vi "clear_buffers.vi"(8 "error in (no error)":errorcluster, 11 "DAQ_DL091205Readers in":refnum<class "DAQ_DL091205Readers.lvclass">) -> (0 "error out":errorcluster, 3 "DAQ_DL091205Readers out":refnum<class "DAQ_DL091205Readers.lvclass">)   [LabVIEW 2010, in "DAQ_DL091205Readers.lvclass"]
uses:
  DAQ_DL091205Readers.lvclass
  DAQ_DL090211Scaffold/DAQ_DL090211Scaffold/DAQ_DL090211Scaffold.lvclass
  DAQ_DL091205Readers.lvclass/DAQ_DL091205Readers.ctl
  SignalReader/GenericSignalReader/GenericSignalReader/GenericSignalReader.lvclass
  common/classes/ErrorController/ErrorController/class_data.vi
  common/classes/ErrorController/ErrorController/ErrorController.lvclass
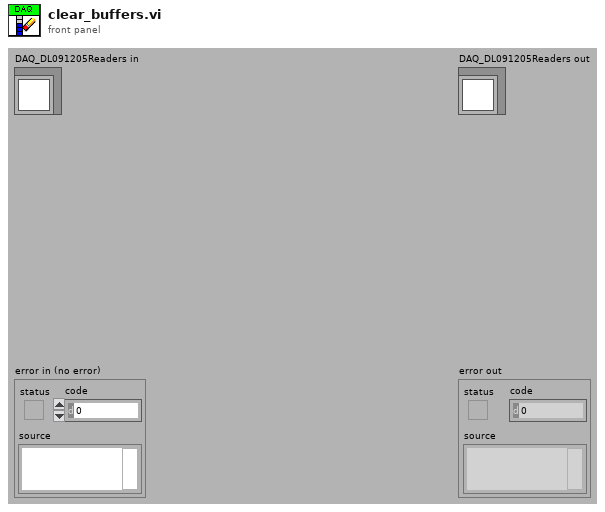
[diagram p1: front panel]
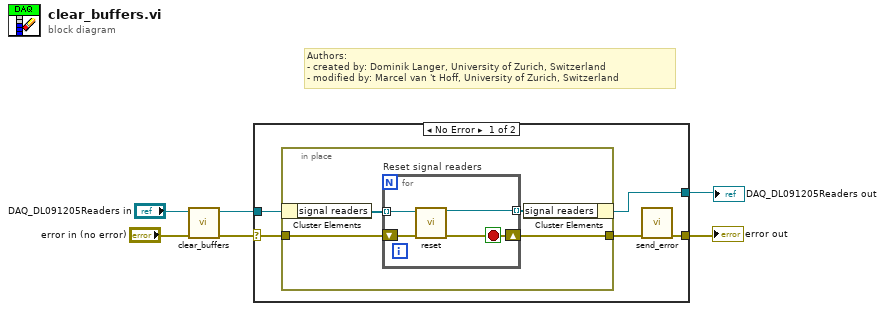
[diagram p0: block diagram]
diagram:
  # "Authors: \n- created by: Dominik Langer, University of Zurich, Switzerland\n- modified by: Marcel van 't Hoff, University of Zurich, Switzerland"
  n1 = call-parent "clear_buffers.vi"("error in (no error)"="error in (no error)", "GenericDAQ in"="DAQ_DL091205Readers in") -> ("error out"=w4:errorcluster, "GenericDAQ out"=w3:refnum<class "DAQ_DL091205Readers.lvclass">)  [unwired: 8 in]
  n2 = case shown="No Error" w4 {
    selector: w4 -> [w11 w20]
    tunnel: w3 -> [w8 w21]
    tunnel: [w7 w21] -> w2
    tunnel: [w10 w20] -> w1
    frame No Error {
      n3 = in-place {
        in-place-border: w11 -> [w15]
        in-place-border: [w14] -> w9
        n4 = in-place-cluster #1(w8) -> ("signal readers"=w13:refnum<class "GenericSignalReader.lvclass">[])
        n5 = for "Reset signal readers" {
          tunnel: w13 -> [w17] mode=indexing
          tunnel: [w19] -> w12 mode=indexing
          shift-right: [w16] -> w14
          shift-left: w15 -> [w18]
          stop <- w16 stop-if-true
          n6 = call-dynamic "reset.vi"("error in (no error)"=w18, "GenericSignalReader in"=w17) -> ("error out"=w16:errorcluster, "GenericSignalReader out"=w19:refnum<class "GenericSignalReader.lvclass">)  [unwired: 8 in]
        }
        n7 = in-place-cluster #1("signal readers"=w12) -> (w7:refnum<class "DAQ_DL091205Readers.lvclass">)
      }
      n8 = call "send_error.vi"("error in (no error)"=w9) -> ("error out"=w10:errorcluster)  [unwired: 10 in]
    }
    frame Error {
    }
  }
  "error out" <- w1
  "DAQ_DL091205Readers out" <- w2
